vi "Test DVR Flatten.vi"() -> ()   [LabVIEW 2021]
uses:
  CIF_NIChn_DAQ_Base.lvclass
  Typedef/Datatype Waveform Channel.ctl
panel:
  out "Array":T1[](array[typedef])
  out "error out":errorcluster
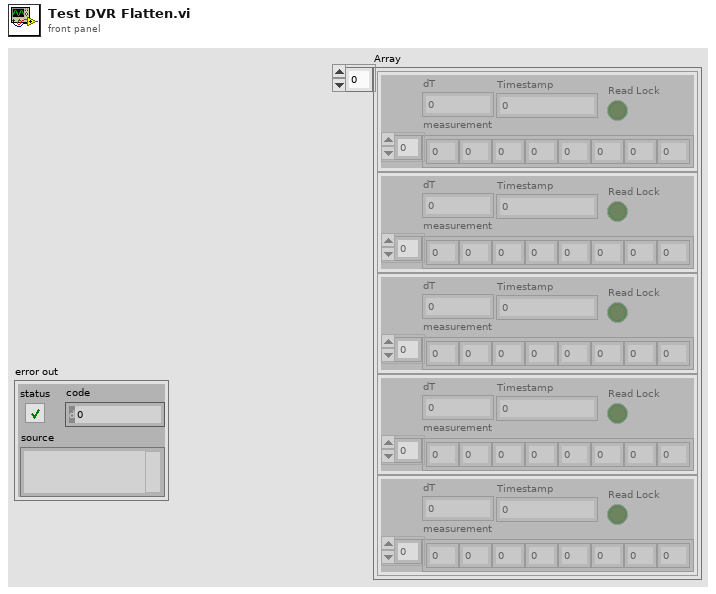
[diagram p1: front panel]
types:
  T1 = typedef "CIF_NIChn_DAQ_Base.lvclass/Datatype Waveform Channel.ctl" = cluster{"measurement":dbl[], "dT":dbl, "Timestamp":i64, "Read Lock":bool}
  T2 = typedef "ChannelCommon.lvlib/Datatype Waveform.ctl" = cluster{"measurement":dbl[], "dT":dbl, "Timestamp":i64, "Read Lock":bool}
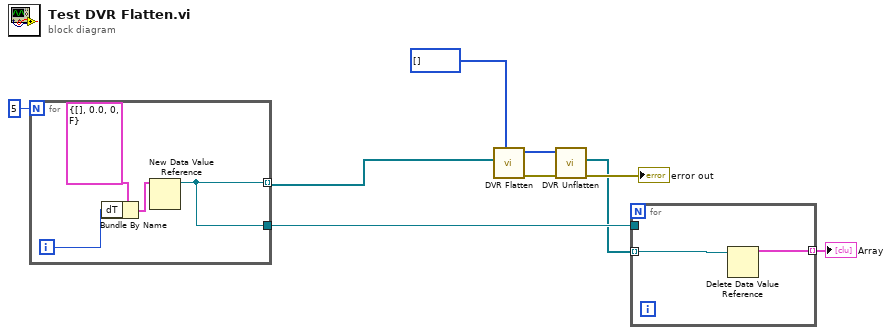
[diagram p0: block diagram]
diagram:
  n1 = for {
    N: 5 -> [_]
    tunnel: [w13] -> w2 mode=indexing
    tunnel: [w13] -> w4
    i -> [w11]
    n2 = Bundle By Name(cluster=T1 {"measurement"=[], "dT"=0.0, "Timestamp"=0, "Read Lock"=FALSE} ("Waveform Datatype"), "dT"=w11) -> (w10:T1)
    n3 = New Data Value Reference(data value=w10) -> (data value reference=w13:refnum<data-value>)  [unwired: 1 in, 1 out]
  }
  n4 = call "DVR Flatten.vi"("payload in"=u8[] [], "Data In"=w2) -> ("error out"=w9:errorcluster, "payload out"=w8:u8[])  [unwired: 5 in, 3 out]
  n5 = call "DVR Unflatten.vi"("error in (no error)"=w9, "Flatten Data in"=w8) -> ("error out"=→"error out":errorcluster, "DVRs Out"=w3:refnum<data-value>[])  [unwired: 6 in, 2 out]
  n6 = for {
    tunnel: w3 -> [w14] mode=indexing
    tunnel: w4 -> [_]
    tunnel: [w15] -> w1 mode=indexing
    n7 = Delete Data Value Reference(data value reference=w14) -> (data value=w15:T2)  [unwired: 1 in, 1 out]
  }
  "Array" <- w1
